vi "TwoTanks (SubVI).vi"(2 "H20 [cm]":dbl, 3 "H10 [cm]":dbl, 4 "Pump On/Off":bool, 5 "Valve1 On/Off":bool, 6 "C2":dbl=35.0, 7 "C1":dbl=32.0, 8 "qmax [cm3/s]":dbl=200.0, 9 "Valve2 On/Off":bool) -> (0 "H2 [cm]":dbl, 1 "H1 [cm]":dbl)   [LabVIEW 2020]
uses:
  <vilib>/Simulation/Implementation/Shared/SIMSCR Execution Mode.ctl
  <vilib>/Simulation/Scripting/Companion Diagram/SimConfigNode/SimParams.ctl
  <vilib>/Simulation/Scripting/Companion Diagram/SimConfigNode/_simSolvers.ctl
  <vilib>/Simulation/Param Hierarchy/Typedefs/SIMPH Param Control Actions.ctl
  <vilib>/Simulation/Implementation/Shared/SIM limit type.ctl
  <vilib>/Simulation/Implementation/Shared/NILVSim_ParamChanged.vi
  <vilib>/Simulation/Implementation/Shared/NILVSIM_BeginStep.vi
  <vilib>/Simulation/DiscreteLinear/Implementation/NILVSim Discrete ZOH.llb/SIM Discrete ZOH (scalar).vi
  <vilib>/Simulation/ContinuousLinear/Implementation/NILVSim Integrator new.llb/SIM Integrator distributor (scalar).vi
  <vilib>/Simulation/SignalArithmetic/Implementation/NILVSim Gain.llb/SIM Gain (scalar).vi
  <vilib>/Simulation/ContinuousLinear/Implementation/NILVSim Integrator new.llb/SIM Integrator collector (scalar).vi
  <vilib>/Simulation/Implementation/Shared/NILVSim_Manager.vi
  <vilib>/Utility/error.llb/Clear Errors.vi
  <vilib>/Simulation/Implementation/Shared/NILVSim_FinalizeModel.vi
  <vilib>/Simulation/Implementation/Shared/SIM Unbundle Sim Info.vi
  <vilib>/Simulation/Implementation/Shared/SIMSH Read Queue.vi
  <vilib>/Simulation/Implementation/Shared/NILVSim_Initialize.vi
  <vilib>/Simulation/Utility/Implementation/NILVSim Get Time and IsAcceptedStep.vi
  <vilib>/Simulation/Implementation/Shared/NILVSim_GetModelError.vi
  <vilib>/Simulation/Implementation/Shared/SIM SimErrorHandler.vi
  <vilib>/Simulation/Implementation/Shared/SIM Bundle Sim Info.vi
  <vilib>/Simulation/Scripting/Companion Diagram/SimConfigNode/SimDog.xnode
  <vilib>/Simulation/Implementation/XNodeFramework/SimXNode/SimX.xnode
  <vilib>/Simulation/ContinuousLinear/Implementation/NILVSim Integrator new.llb/SIM Integrator (scalar).vi
  <vilib>/Simulation/Implementation/Shared/NI_SIM_Implementation.lvlib
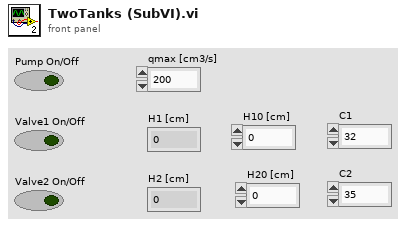
[diagram p1: front panel]
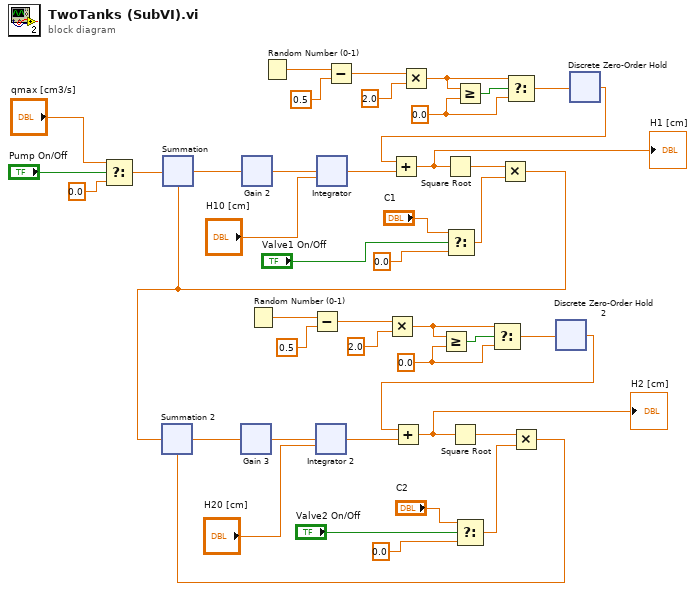
[diagram p0: block diagram]
diagram:
  w5 = 0.0 ("y 6")
  w17 = 0.0 ("y 3")
  n1 = Select ("Select 2")(t="qmax [cm3/s]", s="Pump On/Off", f=0.0 ("f 2")) -> (s? t:f=w34:dbl)
  n2 = Random Number (0-1) ("Random Number (0-1) 2")() -> (number: 0 to 1=w11:dbl)
  n3 = Random Number (0-1)() -> (number: 0 to 1=w24:dbl)
  n4 = Subtract ("Subtract 2")(x=w11, y=0.5 ("y 4")) -> (x-y=w10:dbl)
  n5 = Subtract(x=w24, y=0.5) -> (x-y=w23:dbl)
  n6 = Multiply ("Multiply 4")(x=w10, y=2.0 ("y 5")) -> (x*y=w6:dbl)
  n7 = Multiply ("Multiply 3")(x=w23, y=2.0 ("y 2")) -> (x*y=w18:dbl)
  n8 = Greater Or Equal? ("Greater Or Equal? 2")(x=w6, y=w5) -> (x >= y?=w7:bool)
  n9 = Select(t="C1", s="Valve1 On/Off", f=0.0) -> (s? t:f=w38:dbl)
  n10 = Greater Or Equal?(x=w18, y=w17) -> (x >= y?=w19:bool)
  n11 = Select ("Select 3")(t="C2", s="Valve2 On/Off", f=0.0 ("f 3")) -> (s? t:f=w27:dbl)
  n12 = Select ("Select 5")(t=w6, s=w7, f=w5) -> (s? t:f=w4:dbl)
  n13 = Select ("Select 4")(t=w18, s=w19, f=w17) -> (s? t:f=w15:dbl)
  n14 = xnode "Discrete Zero-Order Hold 2"("input"=w4) -> ("output"=w2:dbl)  [unwired: 4 in]
  n15 = xnode "Discrete Zero-Order Hold"("input"=w15) -> ("output"=w16:dbl)  [unwired: 4 in]
  n16 = xnode "Summation 2"("Operand1"=w14, "Operand2"=w13) -> ("Result"=w32:dbl)
  n17 = xnode "Gain 3"("input"=w32) -> ("output"=w33:dbl)  [unwired: 3 in]
  n18 = xnode "Integrator 2"("input"=w33, "initial condition"="H20 [cm]") -> ("output"=w3:dbl)  [unwired: 8 in, 2 out]
  n19 = Add ("Add 2")(x=w2, y=w3) -> (x+y=w1:dbl)
  "H2 [cm]" <- w1
  n20 = Square Root ("Square Root 2")(x=w1) -> (sqrt(x)=w30:dbl)
  n21 = Multiply ("Multiply 2")(x=w30, y=w27) -> (x*y=w13:dbl)
  n22 = xnode "Summation"("Operand1"=w34, "Operand2"=w14) -> ("Result"=w43:dbl)
  n23 = xnode "Gain 2"("input"=w43) -> ("output"=w44:dbl)  [unwired: 3 in]
  n24 = xnode "Integrator"("input"=w44, "initial condition"="H10 [cm]") -> ("output"=w21:dbl)  [unwired: 8 in, 2 out]
  n25 = Add(x=w16, y=w21) -> (x+y=w12:dbl)
  "H1 [cm]" <- w12
  n26 = Square Root(x=w12) -> (sqrt(x)=w41:dbl)
  n27 = Multiply(x=w41, y=w38) -> (x*y=w14:dbl)
